vi "Configure Scan And Rel.vi"(6 "Number Of Scan Points (2)":i32=2, 7 "Rel Mode (T: Off)":bool caption="Rel Mode (T: On)", 8 "Error In (no error)":errorcluster, 9 "Scan Stop Frequency (200.0E+3)":dbl=200000000.0 format="%.2e", 10 "Scan Start Frequency (25.0E+3)":dbl=25000.0 format="%.2e", 11 "VISA Resource Name":refnum<visa-resource-name>) -> (0 "Error Out":errorcluster, 3 "VISA Resource Name Out":refnum<visa-resource-name>)   [LabVIEW 2010, in "Stanford Research 844.lvlib"]
doc: "This VI configures Scan And Rel."
uses:
  <instrlib>/Stanford Research 844/Stanford Research 844.lvlib
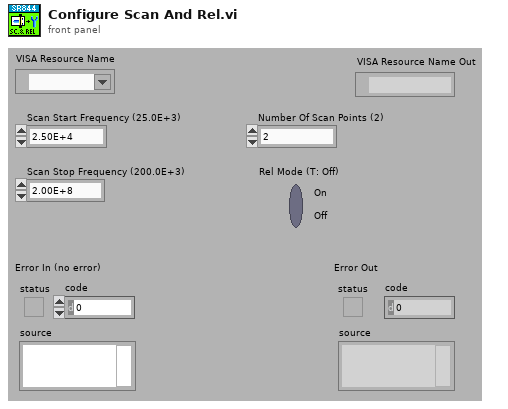
[diagram p1: front panel]
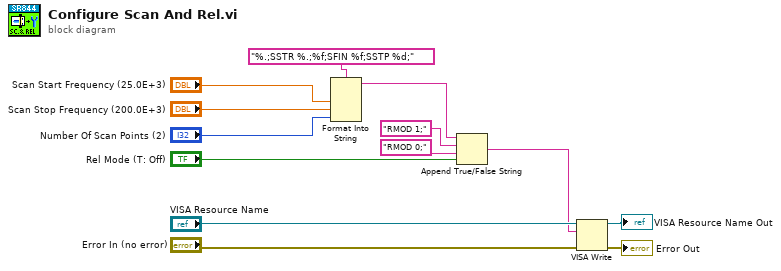
[diagram p0: block diagram]
diagram:
  n1 = Format Into String(format string="%.;SSTR %.;%f;SFIN %f;SSTP %d;", "Scan Start Frequency (25.0E+3)", "Scan Stop Frequency (200.0E+3)", "Number Of Scan Points (2)") -> (resulting string=w5:string)  [unwired: 2 in, 1 out]
  n2 = Append True/False String(1:"Rel Mode (T: Off)", 2:"RMOD 0;" ("true string"), 3:"RMOD 1;" ("true string"), 4:w5) -> (0:w1:string)
  n3 = VISA Write(VISA resource name="VISA Resource Name", write buffer=w1, error in (no error)="Error In (no error)") -> (VISA resource name out=→"VISA Resource Name Out":refnum<visa-resource-name>, error out=→"Error Out":errorcluster)  [unwired: 1 out]
